vi "getStringsArray.vi"(11 "Menu Ring":T1 items=["Guitar", "Ukulele"]) -> (3 "array of frequencies":dbl[](array[numeric]))   [LabVIEW 2019]
uses:
  ChosenInstrument.ctl
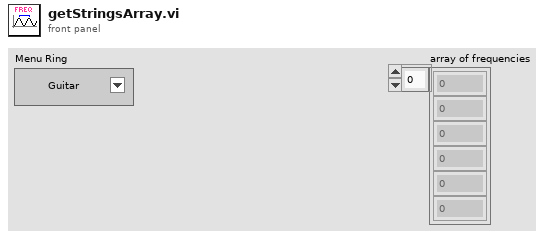
[diagram p1: front panel]
types:
  T1 = typedef "ChosenInstrument.ctl" = u16
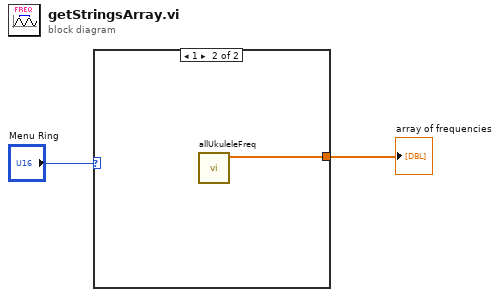
[diagram p0: block diagram]
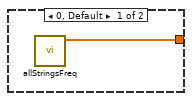
[diagram p2: hidden frame]
diagram:
  n1 = case shown="1" "Menu Ring" {
    tunnel: [w3 w4] -> w1
    frame 0, Default {
      n2 = call "allStringsFreq.vi"() -> ("array of frequencies"=w3:dbl[])  [unwired: 11 in]
    }
    frame 1 {
      n3 = call "allUkuleleFreq.vi"() -> ("array of frequencies"=w4:dbl[])  [unwired: 11 in]
    }
  }
  "array of frequencies" <- w1
